vi "Host_HealthCheck_CompareValue.vi"(10 "Table in":string[][](table) caption="Table Control", 11 "Index":i32) -> (3 "r/g":u32)   [LabVIEW 2018]
doc: "Compares sensor value to listed min/max values and changes cell color in table.\nIN: Index, Updated Table\nOUT: Color"
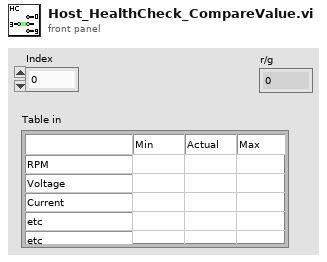
[diagram p1: front panel]
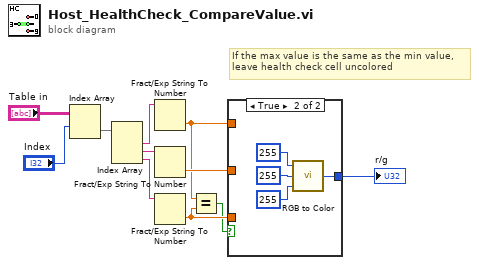
[diagram p0: block diagram]
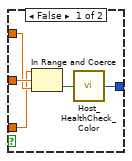
[diagram p2: hidden frame]
diagram:
  # "If the max value is the same as the min value,\nleave health check cell uncolored"
  n1 = Index Array(array="Table in", index (row)="Index") -> (element=w8:string[])  [unwired: 1 in]
  n2 = Index Array(array=w8) -> (element #1=w7:string, element #2=w6:string, element #3=w5:string)  [unwired: 3 in]
  n3 = Fract/Exp String To Number(string=w7) -> (number=w3:dbl)  [unwired: 3 in, 1 out]
  n4 = Fract/Exp String To Number(string=w6) -> (number=w4:dbl)  [unwired: 3 in, 1 out]
  n5 = Fract/Exp String To Number(string=w5) -> (number=w2:dbl)  [unwired: 3 in, 1 out]
  n6 = Equal?(x=w3, y=w2) -> (x = y?=w1:bool)
  n7 = case shown="True" w1 {
    tunnel: [w16 w17] -> w11
    tunnel: w4 -> [w15 _]
    tunnel: w3 -> [w13 _]
    tunnel: w2 -> [w12 _]
    frame False {
      n8 = In Range and Coerce(upper limit=w12, x=w15, lower limit=w13) -> (In Range?=w14:bool)  [unwired: 1 out]
      n9 = call "Host_HealthCheck_Color.vi"("In range?"=w14) -> ("Color out"=w16:u32)
    }
    frame True {
      n10 = call <vilib>:"RGB to Color.vi"("B"=u8 255, "G"=u8 255, "R"=u8 255) -> ("Color"=w17:u32)
    }
  }
  "r/g" <- w11
